vi "Slot Noise Test.vi"   [LabVIEW 2011]
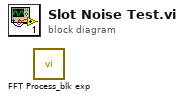
[diagram p0: block diagram]
diagram:
  n1 = call <userlib>:"FFT Process_blk exp.vi"() -> ()  [unwired: 6 in, 6 out]
